vi "Store New Running Function.vi"(8 "error in (no error)":errorcluster, 9 "Caller-To-Actor Enqueuer":refnum<class "Message Enqueuer.lvclass">, 10 "name":string, 11 "Controller in":refnum<class "Controller.lvclass">) -> (0 "error out":errorcluster, 3 "Controller out":refnum<class "Controller.lvclass">)   [LabVIEW 2016, in "Controller Actor.lvlib" / "Controller.lvclass"]
uses:
  <userlib>/Common Components/Controller/Controller.lvclass
  <vilib>/ActorFramework/Message Enqueuer/Message Enqueuer.lvclass
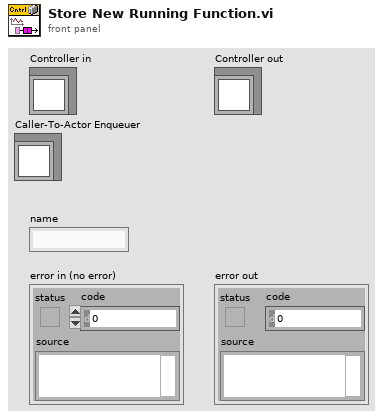
[diagram p1: front panel]
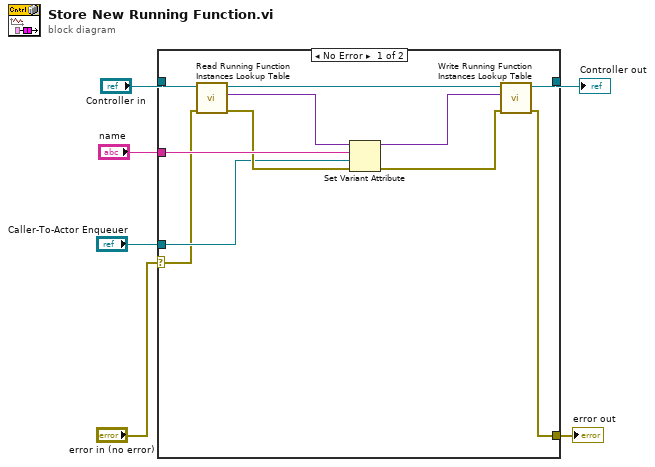
[diagram p0: block diagram]
diagram:
  n1 = case shown="No Error" "error in (no error)" {
    selector: "error in (no error)" -> [w7 w18]
    tunnel: [w17 w18] -> w6
    tunnel: [w14 w19] -> w5
    tunnel: "Controller in" -> [w13 w19]
    tunnel: "name" -> [w12 _]
    tunnel: "Caller-To-Actor Enqueuer" -> [w8 _]
    frame No Error {
      n2 = call <userlib>:"Read Running Function Instances Lookup Table.vi"("error in (no error)"=w7, "Controller in"=w13) -> ("error out"=w10:errorcluster, "Running Function Instances Lookup Table"=w11:variant, "Controller out"=w16:refnum<class "Controller.lvclass">)  [unwired: 7 in]
      n3 = Set Variant Attribute(Variant=w11, name=w12, value=w8, error in=w10) -> (Variant out=w15:variant, error out=w9:errorcluster)  [unwired: 1 out]
      n4 = call <userlib>:"Write Running Function Instances Lookup Table.vi"("error in (no error)"=w9, "Running Function Instances Lookup Table"=w15, "Controller in"=w16) -> ("error out"=w17:errorcluster, "Controller out"=w14:refnum<class "Controller.lvclass">)  [unwired: 7 in]
    }
    frame Error {
    }
  }
  "error out" <- w6
  "Controller out" <- w5
